vi "version.vi"() -> (3 "Version":string)   [LabVIEW 2024]
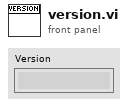
[diagram p1: front panel]
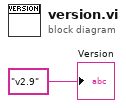
[diagram p0: block diagram]
diagram:
  "Version" <- "v2.9"
